vi "Hormiga_digitalWrite.vi"(8 "error in (no error)":errorcluster, 9 "Value":bool, 10 "Terminal":u8=13, 11 "VISA Refnum in":refnum<visa-resource-name>) -> (0 "error out":errorcluster, 2 "Returned Value":u8, 3 "VISA Refnum out":refnum<visa-resource-name>)   [LabVIEW 2016]
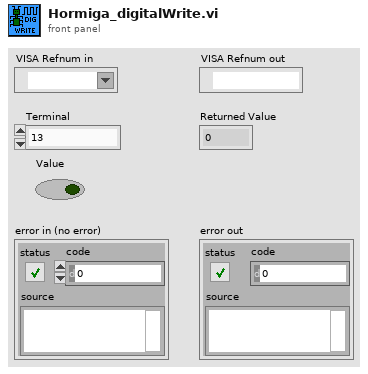
[diagram p1: front panel]
types:
  T1 = enum16{"pinMode", "digitalWrite", "digitalRead", "analogRead", "analogWrite"}
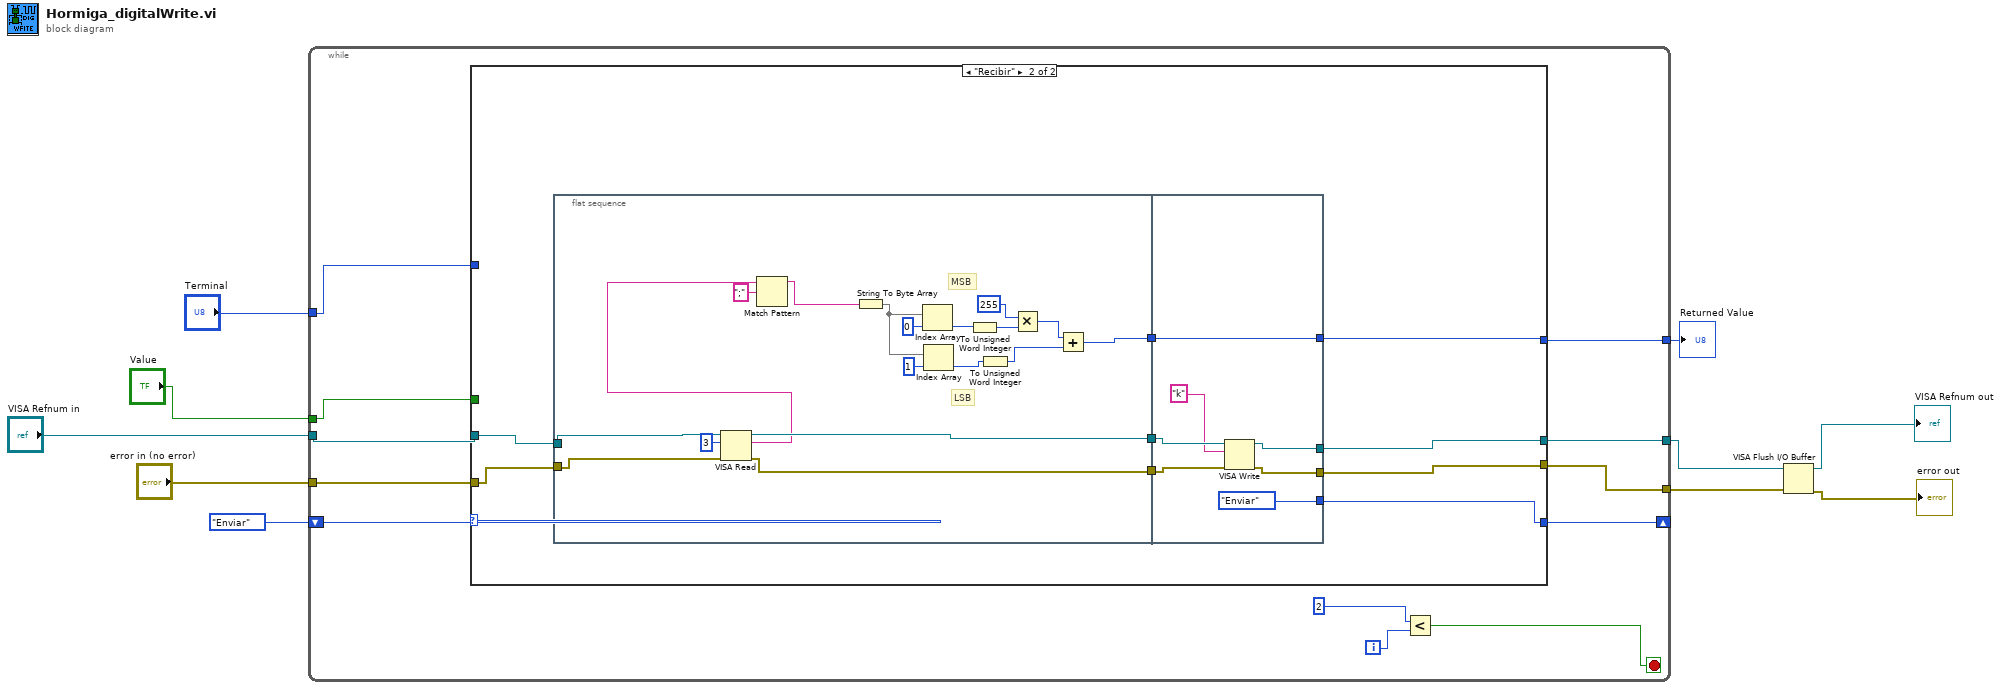
[diagram p0: block diagram]
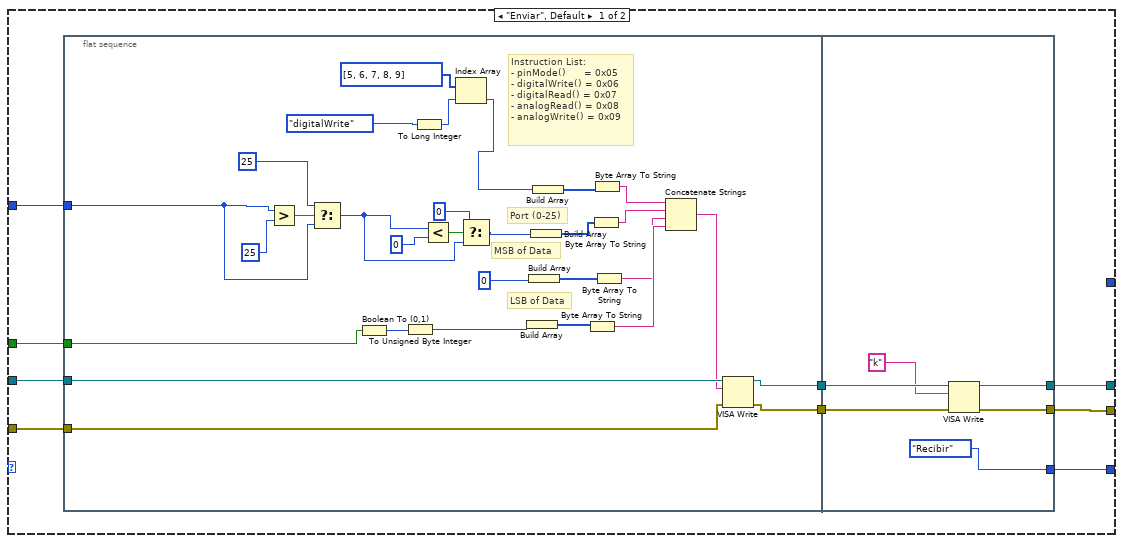
[diagram p2: hidden frame]
diagram:
  n1 = while {
    shift-right: [w17] -> _
    shift-left: enum16{"Enviar", "Recibir"}."Enviar" -> [w22]
    tunnel: "error in (no error)" -> [w21]
    tunnel: "VISA Refnum in" -> [w20]
    tunnel: [w19] -> w4
    tunnel: [w18] -> w3
    tunnel: "Terminal" -> [w13]
    tunnel: "Value" -> [w12]
    tunnel: [w11] -> w10
    i -> [w15]
    stop <- w16 stop-if-true
    n2 = case shown="\"Recibir\"" w22 {
      tunnel: w21 -> [w31 w76]
      tunnel: w20 -> [w30 w75]
      tunnel: [w27 w72] -> w19
      tunnel: [w26 w71] -> w18
      tunnel: [w25 w70] -> w17
      tunnel: w13 -> [w24 _]
      tunnel: w12 -> [w23 _]
      tunnel: [_ w68] -> w11
      frame "Enviar", Default {
        n3 = flat-sequence {
          tunnel: w31 -> [w61]
          tunnel: w30 -> [w60]
          tunnel: [w59] -> w29
          tunnel: [w58] -> w28
          tunnel: w24 -> [w36]
          tunnel: w23 -> [w32]
          tunnel: w29 -> [w67]
          tunnel: w28 -> [w66]
          tunnel: [w64] -> w27
          tunnel: [w63] -> w26
          tunnel: [enum16{"Enviar", "Recibir"}."Recibir"] -> w25
          frame #0 {
            # "Instruction List:\n- pinMode()      = 0x05\n- digitalWrite() = 0x06\n- digitalRead() = 0x07\n- analogRead() = 0x08\n- analogWrite() = 0x09"
            # "LSB of Data"
            # "MSB of Data"
            # "Port (0-25)"
            n4 = Greater?(x=w36, y=u8 25) -> (0:w43:bool)
            n5 = Select(t=u8 25, s=w43, f=w36) -> (s? t:f=w38:u8)
            n6 = Boolean To (0,1)(Boolean=w32) -> (0, 1=w34:i16)
            n7 = To Unsigned Byte Integer(number=w34) -> (unsigned 8bit integer=w33:u8)
            n8 = To Long Integer(number=T1."digitalWrite") -> (32bit integer=w46:i32)
            n9 = Less?(x=w38, y=u8 0) -> (x < y?=w40:bool)
            n10 = Index Array(array=u8[] [5, 6, 7, 8, 9], index=w46) -> (element=w45:u8)
            n11 = Select(t=u8 0, s=w40, f=w38) -> (s? t:f=w37:u8)
            n12 = Build Array(w33) -> (w53:u8[])
            n13 = Build Array(u8 0) -> (w54:u8[])
            n14 = Build Array(w37) -> (w55:u8[])
            n15 = Build Array(w45) -> (w56:u8[])
            n16 = Byte Array To String(unsigned byte array=w53) -> (string=w52:string)
            n17 = Byte Array To String(unsigned byte array=w55) -> (string=w50:string)
            n18 = Byte Array To String(unsigned byte array=w56) -> (string=w49:string)
            n19 = Byte Array To String(unsigned byte array=w54) -> (string=w51:string)
            n20 = Concatenate Strings(w49, w50, w51, w52) -> (w35:string)
            n21 = VISA Write(VISA resource name=w60, write buffer=w35, error in (no error)=w61) -> (VISA resource name out=w58:refnum<visa-resource-name>, error out=w59:errorcluster)  [unwired: 1 out]
          }
          frame #1 {
            n22 = VISA Write(VISA resource name=w66, write buffer="k", error in (no error)=w67) -> (VISA resource name out=w63:refnum<visa-resource-name>, error out=w64:errorcluster)  [unwired: 1 out]
          }
        }
      }
      frame "Recibir" {
        n23 = flat-sequence {
          tunnel: w76 -> [w86]
          tunnel: w75 -> [w85]
          tunnel: [w94] -> w74
          tunnel: [w93] -> w73
          tunnel: [w87] -> w69
          tunnel: w74 -> [w101]
          tunnel: w73 -> [w100]
          tunnel: [w98] -> w72
          tunnel: [w97] -> w71
          tunnel: [enum16{"Enviar", "Recibir"}."Enviar"] -> w70
          tunnel: w69 -> [w95]
          tunnel: [w95] -> w68
          frame #0 {
            # "MSB"
            # "LSB"
            n24 = VISA Read(VISA resource name=w85, byte count=u32 3, error in (no error)=w86) -> (VISA resource name out=w93:refnum<visa-resource-name>, read buffer=w83:string, error out=w94:errorcluster)  [unwired: 1 out]
            n25 = Match Pattern(string=w83, regular expression=";") -> (before substring=w81:string)  [unwired: 1 in, 3 out]
            n26 = String To Byte Array(string=w81) -> (unsigned byte array=w92:u8[])
            n27 = Index Array(array=w92, index=0) -> (element=w80:u8)
            n28 = Index Array(array=w92, index=1) -> (element=w78:u8)
            n29 = To Unsigned Word Integer(number=w80) -> (unsigned 16bit integer=w79:u16)
            n30 = To Unsigned Word Integer(number=w78) -> (unsigned 16bit integer=w77:u16)
            n31 = Multiply(x=u16 255, y=w79) -> (x*y=w89:u16)
            n32 = Add(x=w89, y=w77) -> (x+y=w87:u16)
          }
          frame #1 {
            n33 = VISA Write(VISA resource name=w100, write buffer="k", error in (no error)=w101) -> (VISA resource name out=w97:refnum<visa-resource-name>, error out=w98:errorcluster)  [unwired: 1 out]
          }
        }
      }
    }
    n34 = Less?(x=2, y=w15) -> (x < y?=w16:bool)
  }
  "Returned Value" <- w10
  n35 = VISA Flush I/O Buffer(VISA resource name=w3, error in (no error)=w4) -> (VISA resource name out=→"VISA Refnum out":refnum<visa-resource-name>, error out=→"error out":errorcluster)  [unwired: 1 in]
